vi "MoveNode.vi"(8 "error in":errorcluster, 9 "index":i32, 10 "new parent":T1, 11 "node":T1) -> (0 "error out":errorcluster)   [LabVIEW 2025, in "CEF.lvlib"]
doc: "Moves a node to a new parretn updating the reference in the 3 nodes (child, old parent and new parent).Copyright 2017 National Instruments Corporation\n\nLicensed under the Apache License, Version 2.0 (the \"License\"); you may not use this file except in compliance with the License. You may obtain a copy of the License at http://www.apache.org/licenses/LICENSE-2.0\nUnless required by applicable law or agreed to in writing, software distributed under the License is distributed on an \"AS IS\" BASIS, WITHOUT WARRANTIES OR CONDITIONS OF ANY KIND, either express or implied. See the License for the specific language governing permissions and limitations under the License."
uses:
  CEF.lvlib
  Node/NodeRef.ctl
  Node/CEF_Node.lvclass
  Node/CEF_Node.lvclass/CEF_Node.ctl
  Node/ReadParent.vi
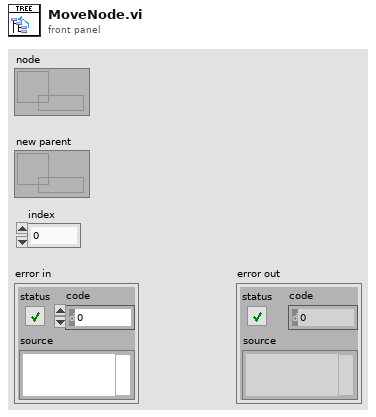
[diagram p1: front panel]
types:
  T1 = typedef "CEF.lvlib/CEF_Node.lvclass/NodeRef.ctl" = refnum<data-value>
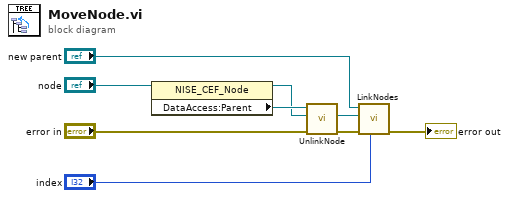
[diagram p0: block diagram]
diagram:
  n1 = property class="NISE_CEF_Node"(reference="node") -> (reference out=w2:T1, "DataAccess:Parent"=w5:T1)  [unwired: 1 in, 1 out]
  n2 = call "UnlinkNode.vi"("error in"="error in", "child in"=w2, "parent in"=w5) -> ("error out"=w4:errorcluster, "child out"=w3:T1)  [unwired: 6 in, 1 out]
  n3 = call "LinkNodes.vi"("index"="index", "error in"=w4, "child in"=w3, "parent in"="new parent") -> ("error out"=→"error out":errorcluster)  [unwired: 5 in, 2 out]
